vi "Check Guest History.vi"(0 "Rooms Manager Model in":refnum<class "Rooms Manager Model.lvclass">, 5 "Guest Contact Number In":string caption="Guest Contact Number", 11 "error in (no error)":errorcluster) -> (4 "Rooms Manager Model out":refnum<class "Rooms Manager Model.lvclass">, 15 "error out":errorcluster)   [LabVIEW 2023, in "Rooms Manager Model.lvlib" / "Rooms Manager Model.lvclass"]
uses:
  Rooms Manager Model.lvclass
  <vilib>/ActorFramework/Actor/Actor.lvclass/Actor.ctl
  Rooms Manager Model.lvclass/Rooms Manager Model.ctl
  Interfaces/Incoming Hotel Management Tool Model Interface Messages/Check Guest History Msg/Check Guest History Msg.lvclass/Check Guest History Msg.ctl
  <vilib>/ActorFramework/Message Enqueuer/Message Enqueuer.lvclass/Message Enqueuer.ctl
  <vilib>/ActorFramework/Message Enqueuer/Enqueue.vi
  Interfaces/Incoming Hotel Management Tool Model Interface Messages/Check Guest History Msg/Check Guest History Msg.lvclass
  <vilib>/ActorFramework/Message Priority Queue/Priority Enqueue.vi
  <vilib>/ActorFramework/Actor/Actor.lvclass
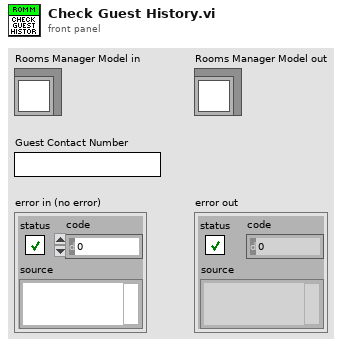
[diagram p1: front panel]
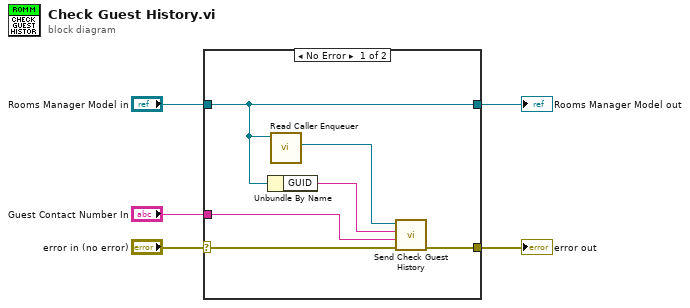
[diagram p0: block diagram]
diagram:
  n1 = case shown="No Error" "error in (no error)" {
    selector: "error in (no error)" -> [w11 w12]
    tunnel: [w10 w12] -> w4
    tunnel: "Guest Contact Number In" -> [w9 _]
    tunnel: "Rooms Manager Model in" -> [w6 w13]
    tunnel: [w6 w13] -> w1
    frame No Error {
      n2 = Unbundle By Name(w6) -> ("GUID"=w7:string)
      n3 = call <vilib>:"Read Caller Enqueuer.vi"("Actor"=w6) -> ("Caller Enqueuer"=w8:refnum<class "Message Enqueuer.lvclass">)  [unwired: 10 in]
      n4 = call "Send Check Guest History.vi"("error in (no error)"=w11, "Guest Contact Number In"=w9, "Rooms Manager GUID"=w7, "Message Enqueuer"=w8) -> ("error out"=w10:errorcluster)  [unwired: 6 in, 1 out]
    }
    frame Error {
    }
  }
  "error out" <- w4
  "Rooms Manager Model out" <- w1
